vi "OAT Calculate Current Speed from Pulse Positions (1 Ch).vi"(7 "reset?":bool, 9 "duration [s]":dbl format="%_6g", 11 "speed position info":T1 {"positions [s]" format="%_6g"}) -> (3 "current speed [RPM]":dbl)   [LabVIEW 2017]
uses:
  <vilib>/addons/Sound and Vibration/Order Analysis/Misc/OAT Position Info.ctl
  <vilib>/addons/_NISVFA/_Shared subVIs/Common/SV Buffer Array (No State) (DBL).vi
  <vilib>/addons/_NISVFA/_Shared subVIs/Common/svc_Get Array Subset (Index).vi
  <vilib>/addons/_NISVFA/_Shared subVIs/Common/svc_Coerce Index and Length.vi
  <vilib>/addons/_NISVFA/_Shared subVIs/Common/svc_Conditional Merge Error.vi
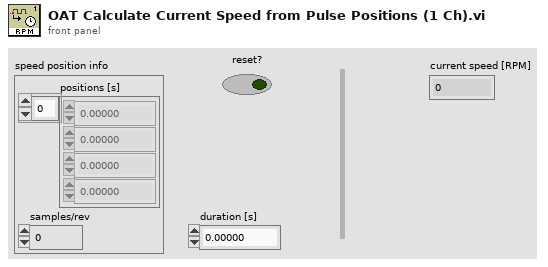
[diagram p1: front panel]
types:
  T1 = typedef "OAT Position Info.ctl" = cluster{"positions [s]":dbl[], "samples/rev":dbl}
  T2 = cluster{"pulse positions":dbl[], "elapsed time":dbl}
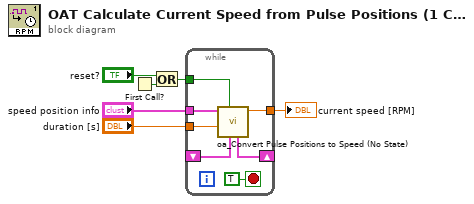
[diagram p0: block diagram]
diagram:
  n1 = First Call?() -> (First Call?: T/F=w3:bool)
  n2 = Or(x="reset?", y=w3) -> (x .or. y?=w1:bool)
  n3 = while {
    tunnel: w1 -> [w7]
    tunnel: "duration [s]" -> [w10]
    shift-right: [w11] -> _
    shift-left: _ -> [w12]
    tunnel: [w8] -> w5
    tunnel: "speed position info" -> [w9]
    stop <- TRUE stop-if-true
    n4 = call <vilib>:"oa_Convert Pulse Positions to Speed (No State).vi"("state in"=w12, "reset?"=w7, "waveform duration"=w10, "speed position info"=w9) -> ("speed [RPM]"=w8:dbl, "state out"=w11:T2)  [unwired: 6 in]
  }
  "current speed [RPM]" <- w5
